vi "MultiByteStrings-Chinese.vi"(8 "Array 2":T1(array[cluster])=[{"String"="管理工具", "String 2"="示例图片", "Cluster"={"String"="远程桌面连接", "Array"=["桌面", "我的文档", "本地磁盘"]}}, {"String"="扫描仪和照相机", "String 2"="示例图片", "Cluster"={"String"="我的电脑", "Array"=["桌面", "画图", "本地磁盘"]}}], 9 "Array":string[](array[string])=["扫描仪和照相机", "计算机管理", "本地安全策略", "事件查看器", "设定程序访问和默认值"], 10 "Cluster":T2={"String"="图片收藏", "String 2"="示例图片", "Cluster"={"String"="我的电脑", "Array"=["桌面", "我的文档", "本地磁盘"]}}, 11 "String":string="新建文件夹") -> ()   [LabVIEW 2009]
panel:
  in  "stop":bool
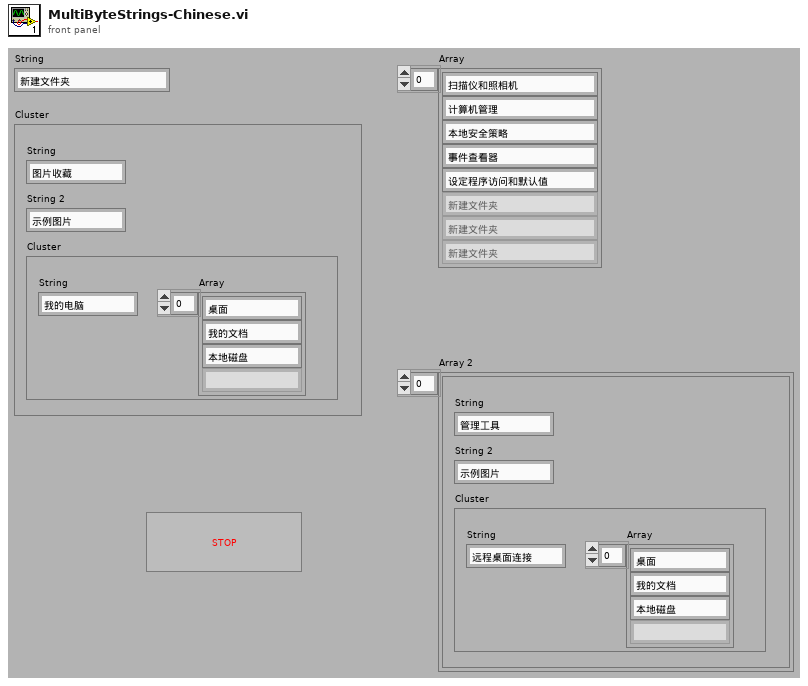
[diagram p1: front panel]
types:
  T1 = cluster{"String":string, "String 2":string, "Cluster":cluster{"String":string, "Array":string[]}}[]
  T2 = cluster{"String":string, "String 2":string, "Cluster":cluster{"String":string, "Array":string[]}}
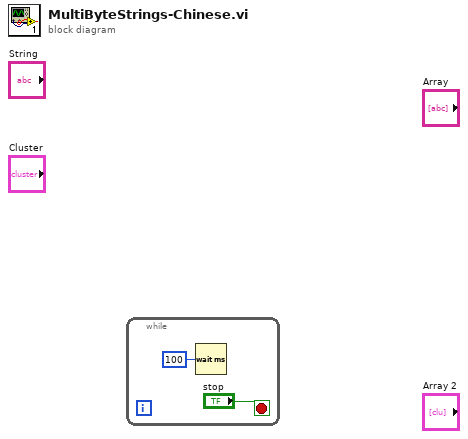
[diagram p0: block diagram]
diagram:
  n1 = while {
    stop <- "stop" stop-if-true
    n2 = Wait (ms)(milliseconds to wait=u32 100) -> ()  [unwired: 1 out]
  }
